vi "Tension Solver.vi"() -> ()   [LabVIEW 2021]
uses:
  <vilib>/Analysis/Matrix/Datatypes/RealMatrix.ctl
  <vilib>/gmath/NumericalOptimization/stopping criteria.ctl
  <vilib>/Platform/TimedLoop/XDataNode/timing_clust.ctl
  <vilib>/Platform/TimedLoop/XDataNode/nitl_modes.ctl
  <vilib>/Platform/TimedLoop/XDataNode/wakeup.ctl
  <vilib>/Analysis/_algsub.llb/Real Vector Norm.vi
  <vilib>/Analysis/baseanly.llb/Real A x B.vi
  <vilib>/Analysis/_algsub.llb/Real PseudoInverse Matrix.vi
  <vilib>/Analysis/Matrix/Numeric/Conversions/Array To Matrix - RA2.vi
  <vilib>/Analysis/Matrix/Numeric/Multiply/Multiply - RM,R.vi
  <vilib>/Analysis/Matrix/Numeric/Conversions/Matrix To Array - RM.vi
  <vilib>/Analysis/Matrix/Numeric/Conversions/Array To Matrix - RA.vi
  <vilib>/gmath/NumericalOptimization/Quadratic Programming AS.vi
  <vilib>/platform/TimedLoop/XDataNode/XDataNode.xnode
  <vilib>/Analysis/NI_AALPro.lvlib
  <vilib>/gmath/NI_Gmath.lvlib
  <vilib>/Analysis/NI_AALBase.lvlib
  <vilib>/Analysis/Matrix/NI_Matrix.lvlib
  <vilib>/Platform/TimedLoop/XDataNode/XDNodeRunTimeDep.lvlib
panel:
  in  "Manual?":bool
  in  "Motor Pos":dbl[][](array[numeric])=[[-2.0, -2.0], [2.0, -2.0], [0.0, 2.0]]
  out "Tension Output":T1(graph)={"Tension[0]"=2.421813674288011, "Tension[1]"=4.109836426279096, "Tension[2]"=-2.2666055322322207, "Tension[3]"=0.0, "Tension[4]"=0.0, "Tension[5]"=0.0, "Tension[6]"=0.0, "Tension[7]"=0.0, "Tension[8]"=0.0}
  in  "Drawing Samples":i32=128
  out "Cluster":T2={"Sim Time"=22.57, "X"=-1.024307661587493, "Y"=0.029017898028761056, "Tension"=[2.421813674288011, 4.109836426279096, -2.2666055322322207]}
  out "Control Time":dbl=22.58000000000073
  in  "Optimization?":bool
  in  "stopping criteria":T3={"function tolerance"=1e-08, "parameter tolerance"=1000000.0, "max iterations"=10000, "max function calls"=10000, "gradient tolerance"=1000000.0, "max time (sec)"=-1.0}
  in  "R":dbl(slide)=1.0 scale=0.0..2.0
  in  "UB":dbl=1000000.0 format="%#_13g"
  in  "LB":dbl=-1000000.0 format="%#_13g"
  out "minimum":dbl[](array[numeric])
  out "Optimized":bool
  in  "P Gain":dbl[](array[numeric])=[50.0, 50.0]
  out "Ref Tension":dbl[](array[numeric])=[2.390219958343406, 4.174578953229368, -2.2502185619036754]
  out "c":T4=[[-10.509026510636803], [-9.557653838992561], [10.212163924365424]]
  out "Q":T4=[[2.0000000000000004, 0.2948894830594344, -1.9987156983704204], [0.2948894830594344, 2.0, -0.22382057154195537], [-1.9987156983704204, -0.22382057154195537, 2.0000000000000004]]
  out "Jacobian Transpose":dbl[][](array[numeric])=[[-0.43130861788505837, -0.9022044536235015], [0.8287494372952807, -0.5596198443432431], [0.46335890194272955, 0.8861707104110518]]
  out "Pos Output":cluster{dbl[], dbl[]}={[-1.024307661587493], [0.029017898028761056]}
  out "Ref Position":cluster{dbl[], dbl[]}={[-0.9961336091430922], [-0.08785119655165322]}
  in  "Tension Control":dbl[](array[slide])=[32.631578947368425, 30.526315789473685, 28.421052631578945] scale=20.0..70.0
  out "Robot Env":cluster{dbl[], dbl[]}[](graph)=[{[-1.024307661587493], [0.029017898028761056]}, {[-2.0, 2.0, 0.0], [-2.0, -2.0, 2.0]}, {[-0.9961336091430922], [-0.08785119655165322]}, {[1.0, 0.9987954562051724, 0.9951847266721969, 0.989176509964781, 0.9807852804032304, 0.970031253194544, 0.9569403357322088, 0.9415440651830208, 0.9238795325112867, 0.9039892931234433, 0.881921264348355, 0.8577286100002721, 0.8314696123025452, 0.8032075314806449, 0.773010453362737, 0.7409511253549591, 0.7071067811865476, 0.6715589548470183, 0.6343932841636455, 0.5956993044924335, 0.5555702330196023, 0.5141027441932217, 0.4713967368259978, 0.4275550934302822, 0.38268343236508984, 0.33688985339222005, 0.29028467725446233, 0.24298017990326398, 0.19509032201612833, 0.14673047445536175, 0.09801714032956077, 0.049067674327418126, 6.123233995736766e-17, -0.04906767432741801, -0.09801714032956065, -0.14673047445536164, -0.1950903220161282, -0.24298017990326387, -0.29028467725446216, -0.33688985339221994, -0.3826834323650897, -0.42755509343028186, -0.4713967368259977, -0.5141027441932217, -0.555570233019602, -0.5956993044924334, -0.6343932841636454, -0.6715589548470184, -0.7071067811865475, -0.7409511253549589, -0.773010453362737, -0.8032075314806448, -0.8314696123025453, -0.857728610000272, -0.8819212643483549, -0.9039892931234433, -0.9238795325112867, -0.9415440651830207, -0.9569403357322088, -0.970031253194544, -0.9807852804032304, -0.989176509964781, -0.9951847266721968, -0.9987954562051724, -1.0, -0.9987954562051724, -0.9951847266721969, -0.989176509964781, -0.9807852804032304, -0.970031253194544, -0.9569403357322089, -0.9415440651830208, -0.9238795325112868, -0.9039892931234434, -0.881921264348355, -0.8577286100002721, -0.8314696123025455, -0.8032075314806449, -0.7730104533627371, -0.7409511253549591, -0.7071067811865477, -0.6715589548470187, -0.6343932841636459, -0.5956993044924331, -0.5555702330196022, -0.5141027441932218, -0.47139673682599786, -0.4275550934302825, -0.38268343236509034, -0.33688985339221994, -0.29028467725446244, -0.24298017990326412, -0.19509032201612866, -0.1467304744553623, -0.09801714032956045, -0.04906767432741803, -1.8369701987210297e-16, 0.04906767432741766, 0.09801714032956009, 0.14673047445536194, 0.1950903220161283, 0.24298017990326376, 0.29028467725446205, 0.3368898533922196, 0.38268343236509, 0.42755509343028214, 0.4713967368259976, 0.5141027441932216, 0.5555702330196018, 0.5956993044924329, 0.6343932841636456, 0.6715589548470183, 0.7071067811865474, 0.7409511253549589, 0.7730104533627367, 0.803207531480645, 0.8314696123025452, 0.857728610000272, 0.8819212643483548, 0.9039892931234431, 0.9238795325112865, 0.9415440651830208, 0.9569403357322088, 0.970031253194544, 0.9807852804032303, 0.9891765099647809, 0.9951847266721969, 0.9987954562051724], [0.0, 0.049067674327418015, 0.0980171403295606, 0.14673047445536175, 0.19509032201612825, 0.24298017990326387, 0.29028467725446233, 0.33688985339222005, 0.3826834323650898, 0.4275550934302821, 0.47139673682599764, 0.5141027441932217, 0.5555702330196022, 0.5956993044924334, 0.6343932841636455, 0.6715589548470183, 0.7071067811865475, 0.7409511253549591, 0.773010453362737, 0.8032075314806448, 0.8314696123025452, 0.8577286100002721, 0.8819212643483549, 0.9039892931234433, 0.9238795325112867, 0.9415440651830208, 0.9569403357322089, 0.970031253194544, 0.9807852804032304, 0.989176509964781, 0.9951847266721968, 0.9987954562051724, 1.0, 0.9987954562051724, 0.9951847266721969, 0.989176509964781, 0.9807852804032304, 0.970031253194544, 0.9569403357322089, 0.9415440651830208, 0.9238795325112867, 0.9039892931234434, 0.881921264348355, 0.8577286100002721, 0.8314696123025455, 0.8032075314806449, 0.7730104533627371, 0.740951125354959, 0.7071067811865476, 0.6715589548470186, 0.6343932841636455, 0.5956993044924335, 0.5555702330196022, 0.5141027441932218, 0.47139673682599786, 0.42755509343028203, 0.3826834323650899, 0.33688985339222033, 0.2902846772544624, 0.24298017990326407, 0.1950903220161286, 0.1467304744553618, 0.09801714032956083, 0.049067674327417966, 1.2246467991473532e-16, -0.049067674327417724, -0.09801714032956059, -0.14673047445536158, -0.19509032201612836, -0.24298017990326382, -0.2902846772544621, -0.3368898533922201, -0.38268343236508967, -0.4275550934302818, -0.47139673682599764, -0.5141027441932216, -0.555570233019602, -0.5956993044924332, -0.6343932841636453, -0.6715589548470184, -0.7071067811865475, -0.7409511253549589, -0.7730104533627367, -0.803207531480645, -0.8314696123025452, -0.857728610000272, -0.8819212643483549, -0.9039892931234431, -0.9238795325112865, -0.9415440651830208, -0.9569403357322088, -0.970031253194544, -0.9807852804032303, -0.9891765099647809, -0.9951847266721969, -0.9987954562051724, -1.0, -0.9987954562051724, -0.9951847266721969, -0.9891765099647809, -0.9807852804032304, -0.970031253194544, -0.9569403357322089, -0.9415440651830209, -0.9238795325112866, -0.9039892931234433, -0.881921264348355, -0.8577286100002722, -0.8314696123025455, -0.8032075314806453, -0.7730104533627369, -0.7409511253549591, -0.7071067811865477, -0.6715589548470187, -0.6343932841636459, -0.5956993044924332, -0.5555702330196022, -0.5141027441932219, -0.4713967368259979, -0.42755509343028253, -0.3826834323650904, -0.33688985339222, -0.2902846772544625, -0.24298017990326418, -0.19509032201612872, -0.1467304744553624, -0.0980171403295605, -0.04906767432741809]}]
  in  "stop":bool
  # "Settings"
  # "Monitor"
  # "Control"
  # "3"
  # "1"
  # "1"
  # "2"
  # "2"
  # "3"
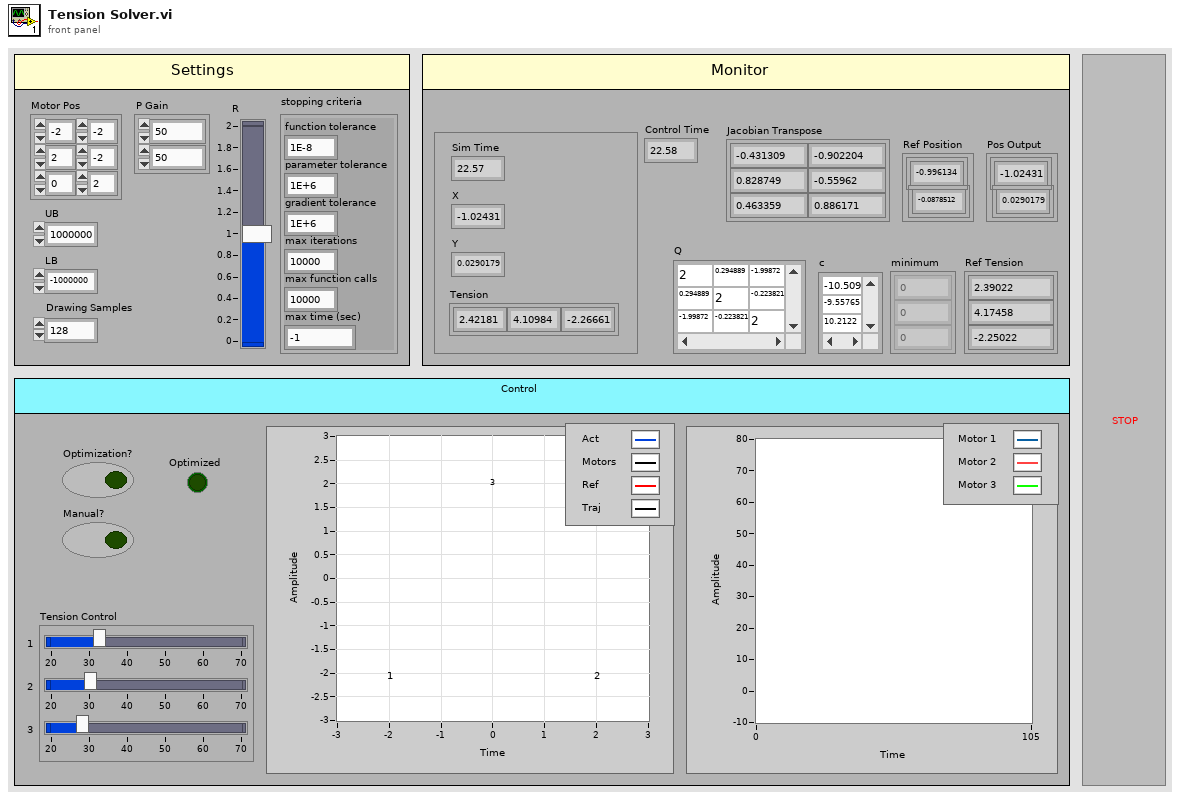
[diagram p1: front panel]
types:
  T1 = cluster{"Tension[0]":dbl, "Tension[1]":dbl, "Tension[2]":dbl, "Tension[3]":dbl, "Tension[4]":dbl, "Tension[5]":dbl, "Tension[6]":dbl, "Tension[7]":dbl, "Tension[8]":dbl}
  T2 = cluster{"Sim Time":dbl, "X":dbl, "Y":dbl, "Tension":dbl[]}
  T3 = typedef "NI_Gmath.lvlib/stopping criteria.ctl" = cluster{"function tolerance":dbl, "parameter tolerance":dbl, "max iterations":i32, "max function calls":i32, "gradient tolerance":dbl, "max time (sec)":dbl}
  T4 = typedef "NI_Matrix.lvlib/RealMatrix.ctl" = dbl[][]
  T5 = typedef "XDNodeRunTimeDep.lvlib/timing_clust.ctl" = cluster{"Expected End [f-1]":u64, "Actual End [f-1]":u64, "Finished Late? [f-1]":bool, "Expected End [i-1]":u64, "Actual End [i-1]":u64, "Finished Late? [i-1]":bool, "Expected Start [i]":u64, "Actual Start [i]":u64, "Expected Start [f]":u64, "Actual Start [f]":u64, "Source Name":string, "Structure Name":string, "Period":i64, "Deadline":i64, "Offset":i64, "Start":i64, "Priority":i32, "Timeout":i32, "Mode":T6, "Wakeup Reason":T7, "Error":errorcluster, "Source Type":string, "Secondary Source Type":string, "Global End Time":u64, "Global Start Time":u64, "Frame Duration":u64, "Iteration Duration":u64, "Assigned CPU":i32, "I/O Scan Engine Mode":u32}
  T6 = typedef "XDNodeRunTimeDep.lvlib/nitl_modes.ctl" = enum32{"No Change", "Process missed periods, maintain original phase", "Discard missed periods, maintain original phase", "Process missed periods, ignore original phase", "Discard missed periods, ignore original phase"}
  T7 = typedef "XDNodeRunTimeDep.lvlib/wakeup.ctl" = enum32{"Normal", "Aborted", "Asynchronous wakeup", "Timing source error", "Timed loop error", "Timeout"}
  T8 = cluster{"Real 2D Array":dbl[][], "Real 2D Array":dbl[]}
  T9 = cluster{"Time":dbl, "X":dbl, "Y":dbl, "Tension":dbl[]}
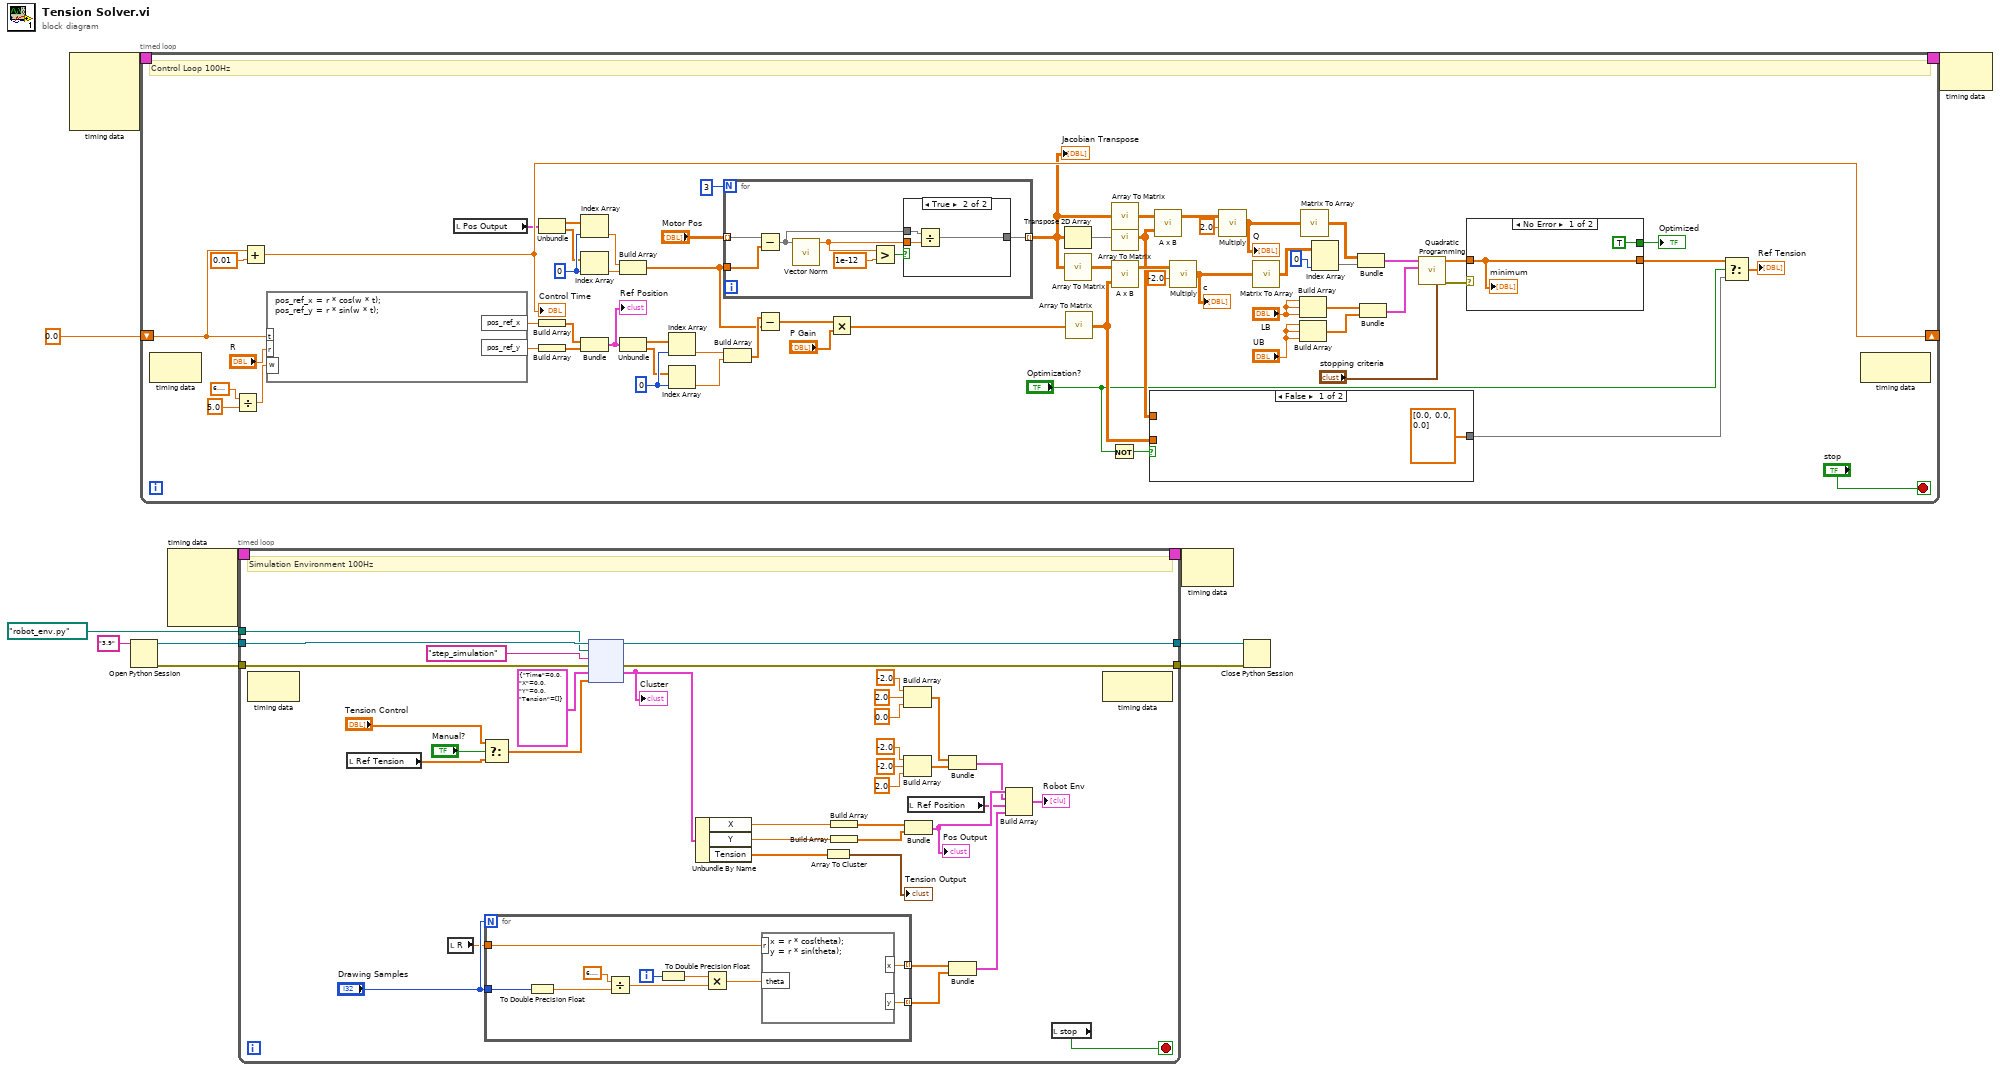
[diagram p0: block diagram]
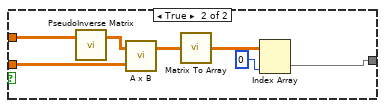
[diagram p2: hidden frame]
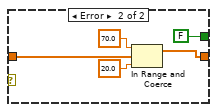
[diagram p3: hidden frame]
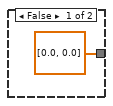
[diagram p4: hidden frame]
diagram:
  n1 = node-c288() -> (w4:T5)  [unwired: 4 in]
  n2 = Open Python Session(python version="3.9" ("Python version")) -> (session out=w6:refnum<k35>, error out=w5:errorcluster)  [unwired: 2 in]
  n3 = timed-loop {
    shift-right: [w68] -> _
    shift-left: 0.0 -> [w69]
    timing: w4 -> [_]
    timing-out: [_] -> w3
    stop <- "stop" stop-if-true
    w55 = 0 ("index")
    w59 = 0 ("index")
    # "Control Loop 100Hz"
    n4 = node-c288() -> ()  [unwired: 1 in, 1 out]
    n5 = Divide(x=6.283185307179586, y=5.0) -> (x/y=w70:dbl)
    n6 = Add(x=w69, y=0.01) -> (x+y=w68:dbl)
    "Control Time" <- w68
    n7 = formula code="pos_ref_x = r * cos(w * t);\npos_ref_y = r * sin(w * t);"("t"=w69, "w"=w70, "r"="R") -> ("pos_ref_y"=w65:dbl, "pos_ref_x"=w66:dbl)
    n8 = local read "Pos Output"() -> (w61:cluster{dbl[], dbl[]})
    n9 = Unbundle(w61) -> (w60:dbl[], w58:dbl[])
    n10 = Build Array(w66) -> (w64:dbl[])
    n11 = Build Array(w65) -> (w63:dbl[])
    n12 = Index Array(array=w60, index=w59) -> (element=w57:dbl)
    n13 = Index Array(array=w58, index=w59) -> (element=w56:dbl)
    n14 = Bundle(w64, w63) -> (w62:cluster{dbl[], dbl[]})  [unwired: 1 in]
    "Ref Position" <- w62
    n15 = Build Array(w57, w56) -> (w28:dbl[])
    n16 = Unbundle(w62) -> (w54:dbl[], w53:dbl[])
    n17 = Index Array(array=w54, index=w55) -> (element=w52:dbl)
    n18 = Index Array(array=w53, index=w55) -> (element=w51:dbl)
    n19 = for {
      N: 3 -> [_]
      tunnel: "Motor Pos" -> [w91] mode=indexing
      tunnel: w28 -> [w93]
      tunnel: [w92] -> w44 mode=indexing
      n20 = Subtract(x=w91, y=w93) -> (x-y=w96:dbl[])
      n21 = call-poly <vilib>:"Vector Norm.vi"("Input Vector"=w96) -> ("norm"=w97:dbl)  [unwired: 9 in, 1 out]
      n22 = Greater?(x=w97, y=1e-12) -> (0:w95:bool)
      n23 = case shown="True" w95 {
        tunnel: w96 -> [_ w101]
        tunnel: w97 -> [_ w100]
        tunnel: [dbl[] [0.0, 0.0] w99] -> w92
        frame False {
        }
        frame True {
          n24 = Divide(x=w101, y=w100) -> (x/y=w99:dbl[])
        }
      }
    }
    "Jacobian Transpose" <- w44
    n25 = Build Array(w52, w51) -> (w29:dbl[])
    n26 = Subtract(x=w29, y=w28) -> (x-y=w27:dbl[])
    n27 = Multiply(x=w27, y="P Gain") -> (x*y=w26:dbl[])
    n28 = Transpose 2D Array(2D array=w44) -> (transposed array=w49:dbl[][])
    n29 = call-poly <vilib>:"Array To Matrix.vi"("Real 2D Array"=w44) -> ("Real Matrix"=w45:T4)
    n30 = call-poly <vilib>:"Array To Matrix.vi"("Real 1D Array"=w26) -> ("Real Matrix (Column Vector)"=w18:T4)
    n31 = Not(x="Optimization?") -> (.not. x?=w16:bool)
    n32 = call-poly <vilib>:"Array To Matrix.vi"("Real 2D Array"=w44) -> ("Real Matrix"=w48:T4)
    n33 = call-poly <vilib>:"Array To Matrix.vi"("Real 2D Array"=w49) -> ("Real Matrix"=w19:T4)
    n34 = call-poly <vilib>:"A x B.vi"("B"=w18, "A"=w45) -> ("A x B"=w42:T4)  [unwired: 1 out]
    n35 = case shown="False" w16 {
      tunnel: w19 -> [_ w77]
      tunnel: w18 -> [_ w76]
      tunnel: [dbl[] [0.0, 0.0, 0.0] ("Real 2D Array") w75] -> w15
      frame False {
      }
      frame True {
        n36 = call-poly <vilib>:"PseudoInverse Matrix.vi"("Input Matrix"=w77) -> ("PseudoInverse Matrix"=w78:T4)  [unwired: 1 in, 1 out]
        n37 = call-poly <vilib>:"A x B.vi"("B"=w76, "A"=w78) -> ("A x B"=w79:T4)  [unwired: 1 out]
        n38 = call-poly <vilib>:"Matrix To Array.vi"("Real Matrix"=w79) -> ("Real 2D Array"=w80:dbl[][])
        n39 = Index Array(array=w80, index (col)=0 ("index")) -> (element=w75:dbl[])  [unwired: 1 in]
      }
    }
    n40 = call-poly <vilib>:"A x B.vi"("B"=w19, "A"=w48) -> ("A x B"=w46:T4)  [unwired: 1 out]
    n41 = call-poly <vilib>:"Multiply.vi"("Real Scalar c"=-2.0 ("y"), "Real Matrix A"=w42) -> ("A * c"=w39:T4)
    "c" <- w39
    n42 = call-poly <vilib>:"Multiply.vi"("Real Scalar c"=2.0 ("y"), "Real Matrix A"=w46) -> ("A * c"=w41:T4)
    "Q" <- w41
    n43 = call-poly <vilib>:"Matrix To Array.vi"("Real Matrix"=w39) -> ("Real 2D Array"=w38:dbl[][])
    n44 = Build Array("LB", "LB", "LB") -> (w33:dbl[])
    n45 = Build Array("UB", "UB", "UB") -> (w32:dbl[])
    n46 = call-poly <vilib>:"Matrix To Array.vi"("Real Matrix"=w41) -> ("Real 2D Array"=w40:dbl[][])
    n47 = Index Array(array=w38, index (col)=0 ("index")) -> (element=w37:dbl[])  [unwired: 1 in]
    n48 = Bundle("Real 2D Array"=w40, "Real 2D Array"=w37) -> (w36:T8)  [unwired: 1 in]
    n49 = Bundle(w33, w32) -> (w31:cluster{dbl[], dbl[]})  [unwired: 1 in]
    n50 = call-poly <vilib>:"Quadratic Programming.vi"("stopping criteria"="stopping criteria", "parameter bounds"=w31, "objective function"=w36) -> ("error out"=w30:errorcluster, "minimum"=w22:dbl[])  [unwired: 5 in, 2 out]
    n51 = case shown="No Error" w30 {
      tunnel: [w84 w87] -> w12
      tunnel: [TRUE ("Boolean") FALSE ("Boolean")] -> w24
      tunnel: w22 -> [w84 w86]
      frame No Error {
        "minimum" <- w84
      }
      frame Error {
        n52 = In Range and Coerce(upper limit=70.0 ("y"), x=w86, lower limit=20.0 ("y")) -> (coerced(x)=w87:dbl[])  [unwired: 1 out]
      }
    }
    "Optimized" <- w24
    n53 = Select(t=w12, s="Optimization?", f=w15) -> (s? t:f=→"Ref Tension":dbl[])
    n54 = node-c288() -> ()  [unwired: 1 in, 1 out]
  }
  n55 = node-c288() -> (w2:T5)  [unwired: 4 in]
  n56 = timed-loop {
    tunnel: w6 -> [w133]
    tunnel: [w136] -> w9
    tunnel: w5 -> [w135]
    tunnel: [w134] -> w7
    tunnel: path "robot_env.py" ("module path") -> [w132]
    timing: w2 -> [_]
    timing-out: [_] -> w1
    stop <- w124 stop-if-true
    # "Simulation Environment 100Hz"
    n57 = node-c288() -> ()  [unwired: 1 in, 1 out]
    n58 = local read "Ref Tension"() -> (w102:dbl[])
    n59 = local read "R"() -> (w106:dbl)
    n60 = Select(t="Tension Control", s="Manual?", f=w102) -> (s? t:f=w103:dbl[])
    n61 = for {
      N: "Drawing Samples" -> [_]
      tunnel: [w149] -> w127 mode=indexing
      tunnel: [w148] -> w126 mode=indexing
      tunnel: "Drawing Samples" -> [w144]
      tunnel: w106 -> [w140]
      i -> [w145]
      n62 = To Double Precision Float(number=w144) -> (double precision float=w142:dbl)
      n63 = Divide(x=6.283185307179586, y=w142) -> (x/y=w147:dbl)
      n64 = To Double Precision Float(number=w145) -> (double precision float=w143:dbl)
      n65 = Multiply(x=w143, y=w147) -> (x*y=w146:dbl)
      n66 = formula code="x = r * cos(theta);\ny = r * sin(theta);"("r"=w140, "theta"=w146) -> ("x"=w149:dbl, "y"=w148:dbl)
    }
    n67 = node(w133, w132, "step_simulation" ("function name"), w135, T9 {"Time"=0.0, "X"=0.0, "Y"=0.0, "Tension"=[]} ("Cluster"), w103) -> (w136:refnum<k35>, w134:errorcluster, w131:T9)  [unwired: 1 in, 2 out]
    "Cluster" <- w131
    n68 = Unbundle By Name(w131) -> ("X"=w113:dbl, "Y"=w111:dbl, "Tension"=w129:dbl[])
    n69 = Array To Cluster(array=w129) -> (cluster=→"Tension Output":T1)
    n70 = Build Array(w113) -> (w112:dbl[])
    n71 = Build Array(w111) -> (w110:dbl[])
    n72 = Build Array(-2.0 ("Y"), 2.0 ("Y"), 0.0 ("Y")) -> (w115:dbl[])
    n73 = Build Array(-2.0 ("Y"), -2.0 ("Y"), 2.0 ("Y")) -> (w114:dbl[])
    n74 = Bundle(w112, w110) -> (w123:cluster{dbl[], dbl[]})  [unwired: 1 in]
    "Pos Output" <- w123
    n75 = local read "Ref Position"() -> (w108:cluster{dbl[], dbl[]})
    n76 = Bundle(w115, w114) -> (w109:cluster{dbl[], dbl[]})  [unwired: 1 in]
    n77 = Bundle(w127, w126) -> (w107:cluster{dbl[], dbl[]})  [unwired: 1 in]
    n78 = Build Array(w123, w109, w108, w107) -> (→"Robot Env":cluster{dbl[], dbl[]}[])
    n79 = local read "stop"() -> (w124:bool)
    n80 = node-c288() -> ()  [unwired: 1 in, 1 out]
  }
  n81 = node-c288(w1) -> ()  [unwired: 1 out]
  n82 = Close Python Session(session in=w9, error in=w7) -> ()  [unwired: 1 out]
  n83 = node-c288(w3) -> ()  [unwired: 1 out]
